vi "AlignmentProc.vi"(8 "error in (no error)":errorcluster, 11 "Refnum in":T2) -> (0 "error out":errorcluster, 1 "Image Dst Out":T1, 2 "Alignment Successful":bool, 3 "Refnum out":T2)   [LabVIEW 2014]
uses:
  <vilib>/userdefined/High Color/VBAIInterface.ctl
  <vilib>/vision/Image Controls.llb/IMAQ Image.ctl
  c_AlignmentProcStates.ctl
  c_VBAI_SelcectInspection.ctl
  c_InstructionEnum.ctl
  c_ReportMessages.ctl
  g_CommandParam.vi
  g_HCCConstants.vi
  g_ImageCalibration.vi
  g_VBAIMeasurements.vi
  g_GPCounters.vi
  g_ReportControl.vi
panel:
  out "Inspection Status":bool
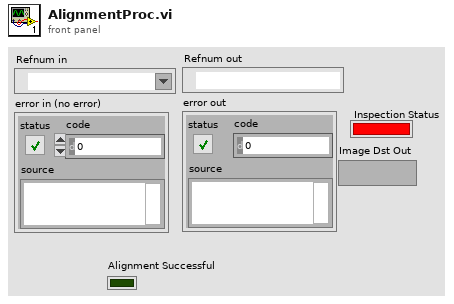
[diagram p1: front panel]
types:
  T1 = typedef "IMAQ Image.ctl" = refnum<image>
  T2 = typedef "VBAIInterface.ctl" = refnum<k21>
  T3 = typedef "c_AlignmentProcStates.ctl" = enum16{"MeasureDistance", "MoveToProbes", "Adjustment", "Fail"}
  T4 = typedef "c_VBAI_SelcectInspection.ctl" = enum16{"Image Acquisition", "Find Reference", "Chip Alignment", "Adjustment", "Porbecard Positioning"}
  T5 = typedef "c_InstructionEnum.ctl" = enum16{"Move Absolute", "Increment", "Move Home", "Motion Kill", "Move Plate", "Set Stepsize", "Query Position"}
  T6 = typedef "c_ReportMessages.ctl" = string
  T7 = cluster{"PASS/FAIL Flag":bool, "Numeric Measurement":dbl, "String Measurement":string, "Report Text":string}
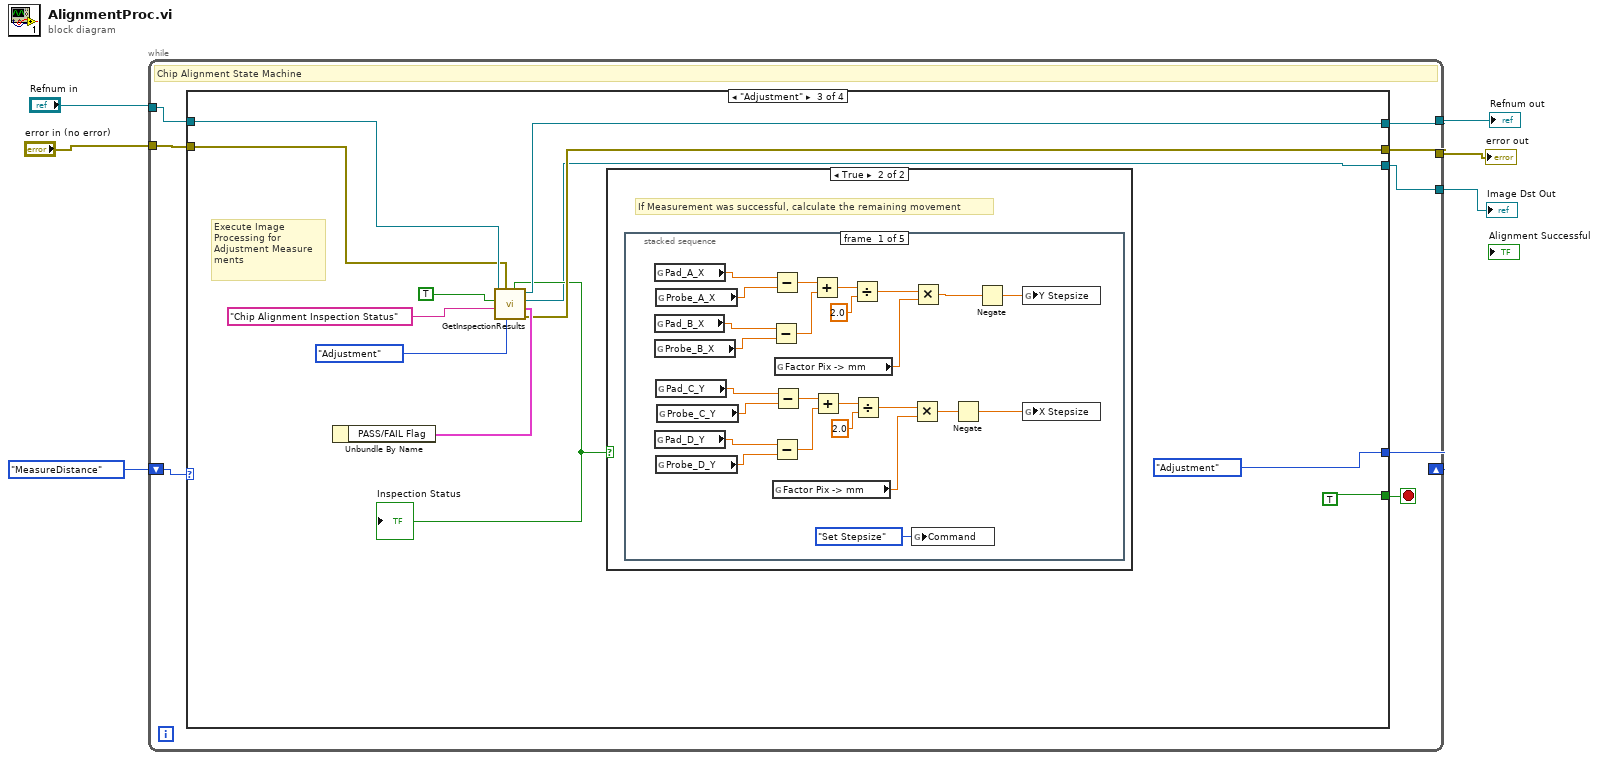
[diagram p0: block diagram]
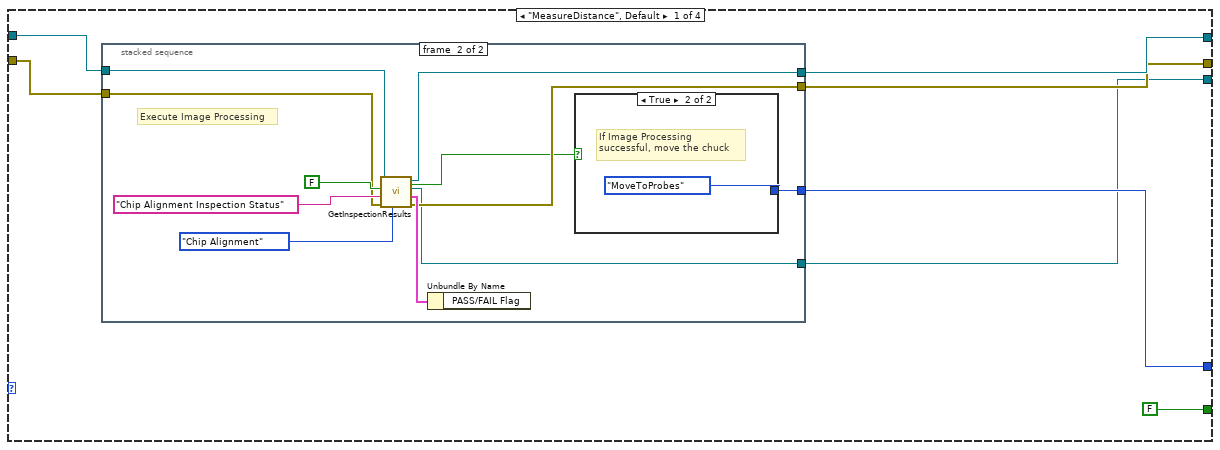
[diagram p2: hidden frame]
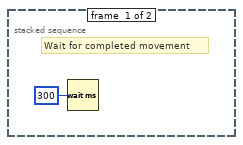
[diagram p3: hidden frame]
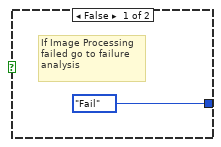
[diagram p4: hidden frame]
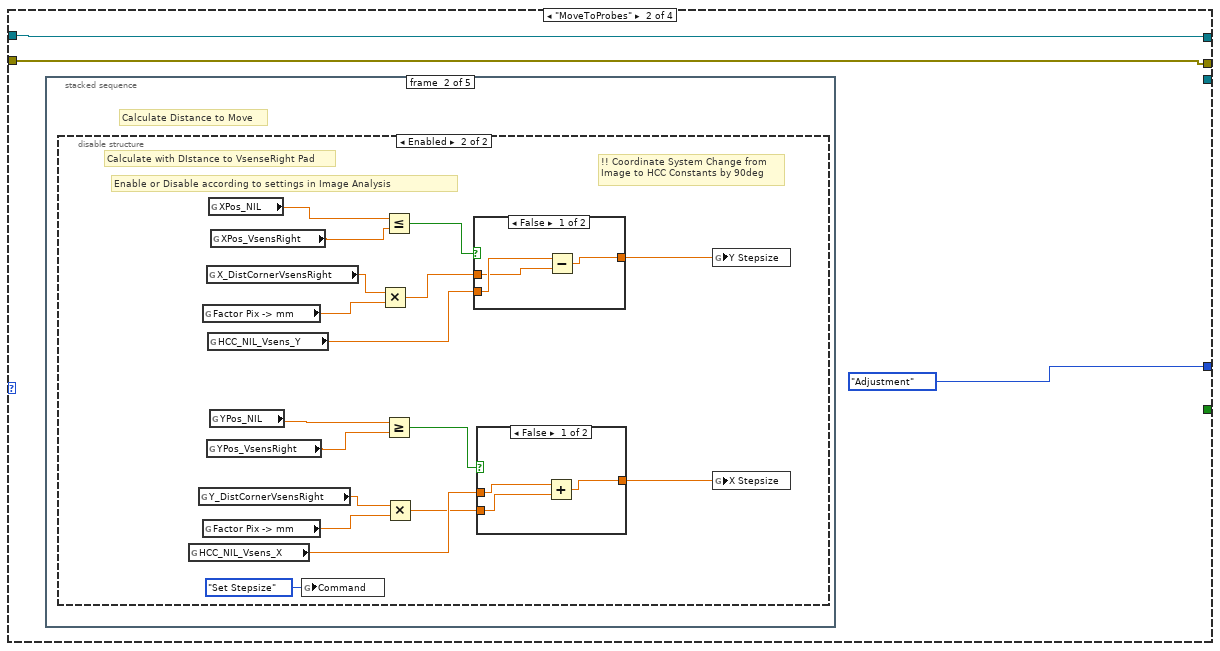
[diagram p5: hidden frame]
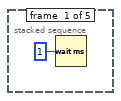
[diagram p6: hidden frame]
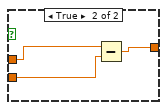
[diagram p8: hidden frame]
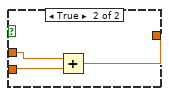
[diagram p9: hidden frame]
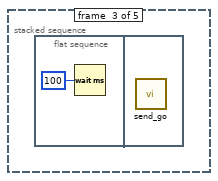
[diagram p10: hidden frame]
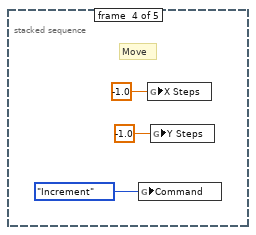
[diagram p11: hidden frame]
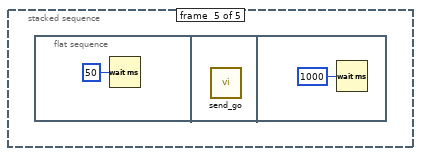
[diagram p12: hidden frame]
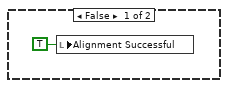
[diagram p13: hidden frame]
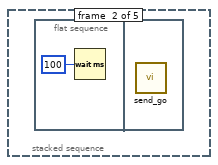
[diagram p14: hidden frame]
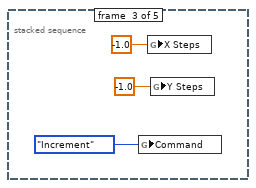
[diagram p15: hidden frame]
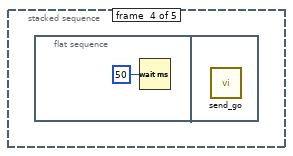
[diagram p16: hidden frame]
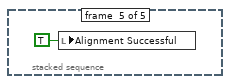
[diagram p17: hidden frame]
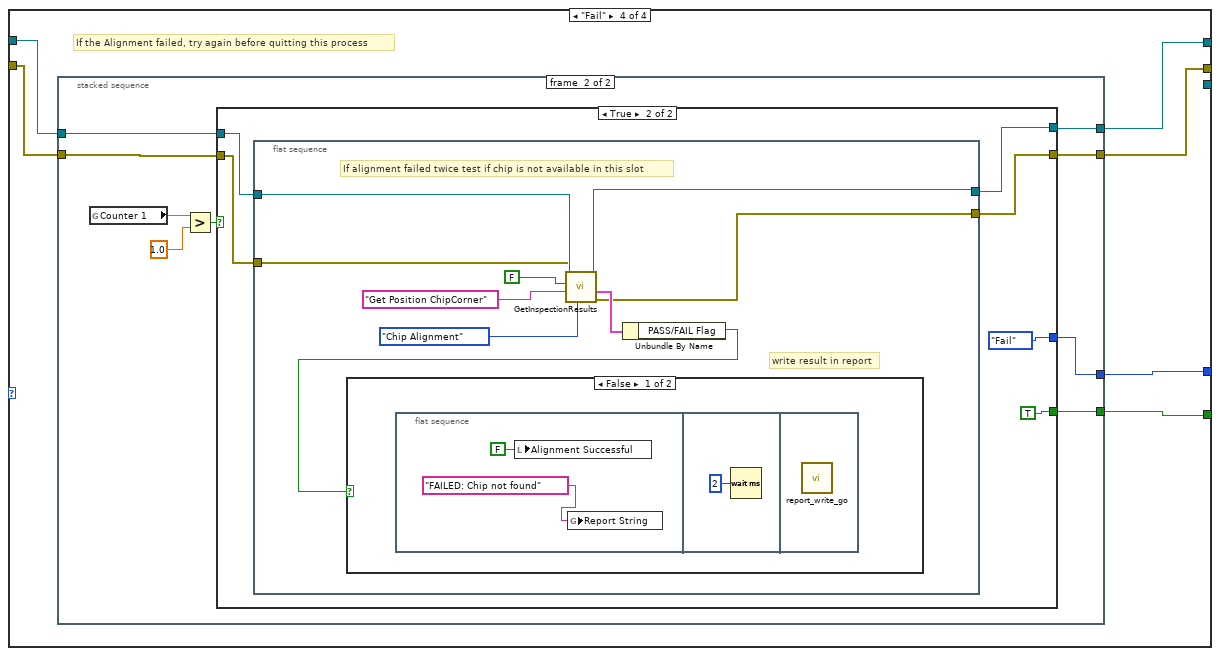
[diagram p18: hidden frame]
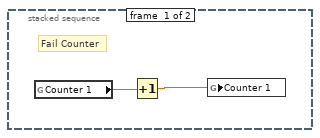
[diagram p19: hidden frame]
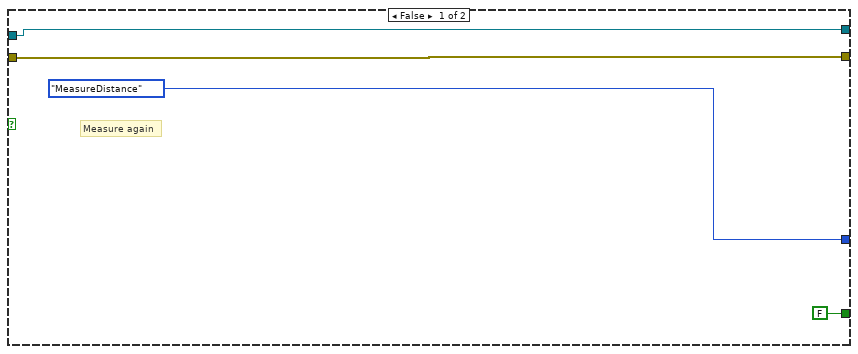
[diagram p20: hidden frame]
diagram:
  n1 = while {
    shift-right: [w10] -> _
    shift-left: c_AlignmentProcStates."MeasureDistance" -> [w14]
    tunnel: [w13] -> w5
    tunnel: [w12] -> w4
    tunnel: "Refnum in" -> [w8]
    tunnel: "error in (no error)" -> [w11]
    tunnel: [w7] -> w1
    stop <- w9 stop-if-true
    # "Chip Alignment State Machine"
    n2 = case shown="\"Adjustment\"" w14 {
      tunnel: [w21 w38 w78 w119] -> w13
      tunnel: [w20 w37 w77 w120] -> w12
      tunnel: w8 -> [w19 w38 w80 w122]
      tunnel: w11 -> [w18 w37 w79 w121]
      tunnel: [w17 c_AlignmentProcStates."Adjustment" c_AlignmentProcStates."Adjustment" w124] -> w10
      tunnel: [FALSE _ TRUE w123] -> w9
      tunnel: [w15 _ w75 _] -> w7
      frame "MeasureDistance", Default {
        n3 = stacked-sequence {
          tunnel: [_ w29] -> w21
          tunnel: [_ w28] -> w20
          tunnel: w19 -> [_ w27]
          tunnel: w18 -> [_ w26]
          tunnel: [_ w25] -> w17
          tunnel: [_ w23] -> w15
          frame #0 {
            # "Wait for completed movement"
            n4 = Wait (ms)(milliseconds to wait=u32 300) -> ()  [unwired: 1 out]
          }
          frame #1 {
            # "Execute Image Processing"
            n5 = call "GetInspectionResults.vi"("Select Inspection"=c_VBAI_SelcectInspection."Chip Alignment", "error in (no error)"=w26, "StepName"="Chip Alignment Inspection Status", "Image Enable"=FALSE, "Refnum in"=w27) -> ("error out"=w28:errorcluster, "Results"=w30:T7, "Image Dst Out"=w23:T1, "Refnum out"=w29:T2, "Inspection Status"=w24:bool)  [unwired: 2 in]
            n6 = Unbundle By Name(w30) -> ()  [unwired: 1 out]
            n7 = case shown="True" w24 {
              tunnel: [c_AlignmentProcStates."Fail" c_AlignmentProcStates."MoveToProbes"] -> w25
              frame False {
                # "If Image Processing\nfailed go to failure \nanalysis"
              }
              frame True {
                # "If Image Processing\nsuccessful, move the chuck"
              }
            }
          }
        }
      }
      frame "MoveToProbes" {
        n8 = stacked-sequence {
          frame #0 {
            n9 = Wait (ms)(milliseconds to wait=u32 1) -> ()  [unwired: 1 out]
          }
          frame #1 {
            # "Calculate Distance to Move"
            n10 = disable-structure shown="Enabled" {
              frame Disabled {
              }
              frame Enabled {
                # "!! Coordinate System Change from\nImage to HCC Constants by 90deg"
                # "Enable or Disable according to settings in Image Analysis"
                # "Calculate with DIstance to VsenseRight Pad"
                n11 = global read "g_HCCConstants.vi" "HCC_NIL_Vsens_X"() -> (w49:dbl)
                n12 = global read "g_VBAIMeasurements.vi" "Y_DistCornerVsensRight"() -> (w42:dbl)
                n13 = global read "g_ImageCalibration.vi" "Factor Pix -> mm"() -> (w55:dbl)
                n14 = global read "g_ImageCalibration.vi" "Factor Pix -> mm"() -> (w54:dbl)
                n15 = global read "g_VBAIMeasurements.vi" "X_DistCornerVsensRight"() -> (w45:dbl)
                n16 = global read "g_VBAIMeasurements.vi" "YPos_VsensRight"() -> (w43:dbl)
                n17 = global read "g_HCCConstants.vi" "HCC_NIL_Vsens_Y"() -> (w51:dbl)
                n18 = global read "g_VBAIMeasurements.vi" "XPos_NIL"() -> (w47:dbl)
                n19 = global read "g_VBAIMeasurements.vi" "YPos_NIL"() -> (w44:dbl)
                n20 = global read "g_VBAIMeasurements.vi" "XPos_VsensRight"() -> (w46:dbl)
                n21 = global write "g_CommandParam.vi" "Command"(c_InstructionEnum."Set Stepsize" ("Command")) -> ()
                n22 = Multiply(x=w45, y=w55) -> (x*y=w52:dbl)
                n23 = Less Or Equal?(x=w47, y=w46) -> (x <= y?=w53:bool)
                n24 = Greater Or Equal?(x=w44, y=w43) -> (x >= y?=w50:bool)
                n25 = Multiply(x=w42, y=w54) -> (x*y=w48:dbl)
                n26 = case shown="False" w53 {
                  tunnel: w52 -> [w64 w68]
                  tunnel: w51 -> [w65 w67]
                  tunnel: [w63 w66] -> w41
                  frame False {
                    n27 = Subtract(x=w65, y=w64) -> (x-y=w63:dbl)
                  }
                  frame True {
                    n28 = Add(x=w68, y=w67) -> (x+y=w66:dbl)
                  }
                }
                n29 = case shown="False" w50 {
                  tunnel: w49 -> [w59 w62]
                  tunnel: w48 -> [w58 w61]
                  tunnel: [w57 w60] -> w40
                  frame False {
                    n30 = Add(x=w59, y=w58) -> (x+y=w57:dbl)
                  }
                  frame True {
                    n31 = Subtract(x=w62, y=w61) -> (x-y=w60:dbl)
                  }
                }
                n32 = global write "g_CommandParam.vi" "Y Stepsize"(w41) -> ()
                n33 = global write "g_CommandParam.vi" "X Stepsize"(w40) -> ()
              }
            }
          }
          frame #2 {
            n34 = flat-sequence {
              frame #0 {
                n35 = Wait (ms)(milliseconds to wait=u32 100) -> ()  [unwired: 1 out]
              }
              frame #1 {
                n36 = call "send_go.vi"() -> ()  [unwired: 12 in]
              }
            }
          }
          frame #3 {
            # "Move"
            n37 = global write "g_CommandParam.vi" "Command"(c_InstructionEnum."Increment" ("Command")) -> ()
            n38 = global write "g_CommandParam.vi" "X Steps"(-1.0 ("Y Stepsize")) -> ()
            n39 = global write "g_CommandParam.vi" "Y Steps"(-1.0 ("Y Stepsize")) -> ()
          }
          frame #4 {
            n40 = flat-sequence {
              frame #0 {
                n41 = Wait (ms)(milliseconds to wait=u32 50) -> ()  [unwired: 1 out]
              }
              frame #1 {
                n42 = call "send_go.vi"() -> ()  [unwired: 12 in]
              }
              frame #2 {
                n43 = Wait (ms)(milliseconds to wait=u32 1000) -> ()  [unwired: 1 out]
              }
            }
          }
        }
      }
      frame "Adjustment" {
        # "Execute Image\nProcessing for\nAdjustment Measure\nments"
        n44 = call "GetInspectionResults.vi"("Select Inspection"=c_VBAI_SelcectInspection."Adjustment", "error in (no error)"=w79, "StepName"="Chip Alignment Inspection Status", "Image Enable"=TRUE, "Refnum in"=w80) -> ("error out"=w77:errorcluster, "Results"=w81:T7, "Image Dst Out"=w75:T1, "Refnum out"=w78:T2, "Inspection Status"=w76:bool)  [unwired: 2 in]
        "Inspection Status" <- w76
        n45 = Unbundle By Name(w81) -> ()  [unwired: 1 out]
        n46 = case shown="True" w76 {
          frame False {
            n47 = local write "Alignment Successful"(TRUE ("Alignment Successful")) -> ()
          }
          frame True {
            # "If Measurement was successful, calculate the remaining movement"
            n48 = stacked-sequence {
              frame #0 {
                n49 = global read "g_VBAIMeasurements.vi" "Pad_A_X"() -> (w112:dbl)
                n50 = global read "g_VBAIMeasurements.vi" "Pad_B_X"() -> (w110:dbl)
                n51 = global read "g_VBAIMeasurements.vi" "Probe_B_X"() -> (w109:dbl)
                n52 = global read "g_VBAIMeasurements.vi" "Pad_D_Y"() -> (w99:dbl)
                n53 = global read "g_VBAIMeasurements.vi" "Probe_A_X"() -> (w111:dbl)
                n54 = global read "g_VBAIMeasurements.vi" "Pad_C_Y"() -> (w97:dbl)
                n55 = global read "g_VBAIMeasurements.vi" "Probe_D_Y"() -> (w100:dbl)
                n56 = global read "g_VBAIMeasurements.vi" "Probe_C_Y"() -> (w98:dbl)
                n57 = Subtract(x=w110, y=w109) -> (x-y=w107:dbl)
                n58 = Subtract(x=w112, y=w111) -> (x-y=w108:dbl)
                n59 = Subtract(x=w99, y=w100) -> (x-y=w102:dbl)
                n60 = Subtract(x=w97, y=w98) -> (x-y=w101:dbl)
                n61 = global read "g_ImageCalibration.vi" "Factor Pix -> mm"() -> (w91:dbl)
                n62 = global read "g_ImageCalibration.vi" "Factor Pix -> mm"() -> (w94:dbl)
                n63 = Add(x=w108, y=w107) -> (x+y=w106:dbl)
                n64 = Add(x=w101, y=w102) -> (x+y=w103:dbl)
                n65 = Divide(x=w106, y=2.0) -> (x/y=w95:dbl)
                n66 = Divide(x=w103, y=2.0) -> (x/y=w92:dbl)
                n67 = Multiply(x=w92, y=w91) -> (x*y=w90:dbl)
                n68 = global write "g_CommandParam.vi" "Command"(c_InstructionEnum."Set Stepsize" ("Command")) -> ()
                n69 = Multiply(x=w95, y=w94) -> (x*y=w93:dbl)
                n70 = Negate(x=w90) -> (-x=w89:dbl)
                n71 = Negate(x=w93) -> (-x=w88:dbl)
                n72 = global write "g_CommandParam.vi" "Y Stepsize"(w88) -> ()
                n73 = global write "g_CommandParam.vi" "X Stepsize"(w89) -> ()
              }
              frame #1 {
                n74 = flat-sequence {
                  frame #0 {
                    n75 = Wait (ms)(milliseconds to wait=u32 100) -> ()  [unwired: 1 out]
                  }
                  frame #1 {
                    n76 = call "send_go.vi"() -> ()  [unwired: 12 in]
                  }
                }
              }
              frame #2 {
                n77 = global write "g_CommandParam.vi" "Command"(c_InstructionEnum."Increment" ("Command")) -> ()
                n78 = global write "g_CommandParam.vi" "X Steps"(-1.0 ("Y Stepsize")) -> ()
                n79 = global write "g_CommandParam.vi" "Y Steps"(-1.0 ("Y Stepsize")) -> ()
              }
              frame #3 {
                n80 = flat-sequence {
                  frame #0 {
                    n81 = Wait (ms)(milliseconds to wait=u32 50) -> ()  [unwired: 1 out]
                  }
                  frame #1 {
                    n82 = call "send_go.vi"() -> ()  [unwired: 12 in]
                  }
                }
              }
              frame #4 {
                n83 = local write "Alignment Successful"(TRUE ("Alignment Successful")) -> ()
              }
            }
          }
        }
      }
      frame "Fail" {
        # "If the Alignment failed, try again before quitting this process"
        n84 = stacked-sequence {
          tunnel: [_ w132] -> w124
          tunnel: [_ w131] -> w123
          tunnel: w122 -> [_ w130]
          tunnel: w121 -> [_ w129]
          tunnel: [_ w128] -> w120
          tunnel: [_ w127] -> w119
          frame #0 {
            # "Fail Counter"
            n85 = global read "g_GPCounters.vi" "Counter 1"() -> (w126:dbl)
            n86 = Increment(x=w126) -> (x+1=w125:dbl)
            n87 = global write "g_GPCounters.vi" "Counter 1"(w125) -> ()
          }
          frame #1 {
            n88 = global read "g_GPCounters.vi" "Counter 1"() -> (w135:dbl)
            n89 = Greater?(x=w135, y=1.0) -> (0:w133:bool)
            n90 = case shown="True" w133 {
              tunnel: [c_AlignmentProcStates."MeasureDistance" c_AlignmentProcStates."Fail"] -> w132
              tunnel: [FALSE TRUE] -> w131
              tunnel: w130 -> [w137 w143]
              tunnel: w129 -> [w136 w142]
              tunnel: [w136 w141] -> w128
              tunnel: [w137 w140] -> w127
              frame False {
                # "Measure again"
              }
              frame True {
                n91 = flat-sequence {
                  tunnel: w143 -> [w150]
                  tunnel: w142 -> [w149]
                  tunnel: [w148] -> w141
                  tunnel: [w147] -> w140
                  frame #0 {
                    # "write result in report"
                    # "If alignment failed twice test if chip is not available in this slot"
                    n92 = call "GetInspectionResults.vi"("Select Inspection"=c_VBAI_SelcectInspection."Chip Alignment", "error in (no error)"=w149, "StepName"="Get Position ChipCorner", "Image Enable"=FALSE, "Refnum in"=w150) -> ("error out"=w148:errorcluster, "Results"=w151:T7, "Refnum out"=w147:T2)  [unwired: 2 in, 2 out]
                    n93 = Unbundle By Name(w151) -> ("PASS/FAIL Flag"=w146:bool)
                    n94 = case shown="False" w146 {
                      frame False {
                        n95 = flat-sequence {
                          frame #0 {
                            n96 = local write "Alignment Successful"(FALSE ("Alignment Successful")) -> ()
                            n97 = global write "g_ReportControl.vi" "Report String"(T6 "FAILED: Chip not found" ("Combo Box")) -> ()
                          }
                          frame #1 {
                            n98 = Wait (ms)(milliseconds to wait=u32 2) -> ()  [unwired: 1 out]
                          }
                          frame #2 {
                            n99 = call "report_write_go.vi"() -> ()  [unwired: 12 in]
                          }
                        }
                      }
                      frame True {
                        n100 = flat-sequence {
                          frame #0 {
                            n101 = local write "Alignment Successful"(FALSE ("Alignment Successful")) -> ()
                            n102 = global write "g_ReportControl.vi" "Report String"(T6 "FAILED: Alignment Process" ("Combo Box")) -> ()
                          }
                          frame #1 {
                            n103 = Wait (ms)(milliseconds to wait=u32 2) -> ()  [unwired: 1 out]
                          }
                          frame #2 {
                            n104 = call "report_write_go.vi"() -> ()  [unwired: 12 in]
                          }
                        }
                      }
                    }
                  }
                }
              }
            }
          }
        }
      }
    }
  }
  "Refnum out" <- w5
  "error out" <- w4
  "Image Dst Out" <- w1
